vi "DecodeRobotsVSSwithOrientation.vi"(5 "offset":i32, 7 "error in (no error)":errorcluster, 8 "array w/ subset deleted in":u8[](array[numeric])) -> (0 "error out":errorcluster, 1 "array w/ subset deleted out":u8[](array[numeric]), 3 "Array":T1[](array[typedef]) {"orientation" format="%+4.3f"; "y" format="%+4.3f"; "confidence" format="%4.3f"; "x" format="%+4.3f"})   [LabVIEW 2017]
uses:
  SSL Detection Robot.ctl
  <vilib>/Analysis/Matrix/Datatypes/RealMatrix.ctl
  <vilib>/Analysis/Matrix/NI_Matrix.lvlib
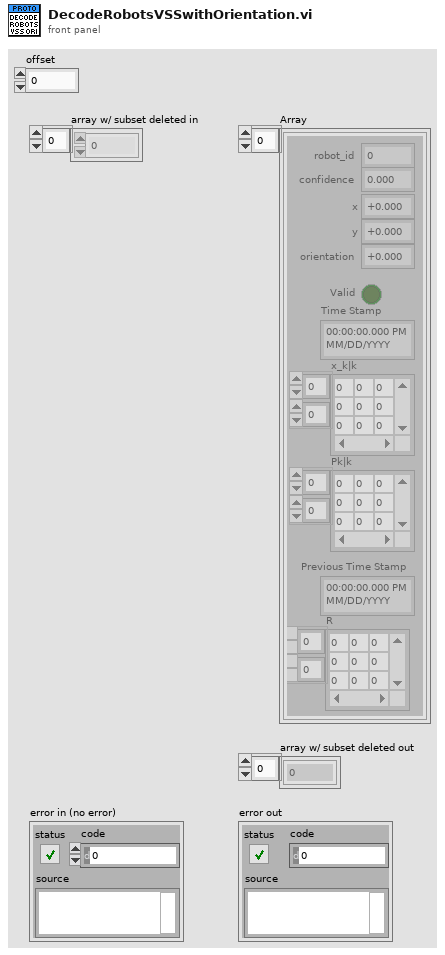
[diagram p1: front panel]
types:
  T1 = typedef "SSL Detection Robot.ctl" = cluster{"x":sgl, "robot_id":u32, "confidence":sgl, "y":sgl, "orientation":sgl, "Valid":bool, "Time Stamp":timestamp, "x_k|k":T2, "Pk|k":T2, "Previous Time Stamp":timestamp, "R":T2}
  T2 = typedef "NI_Matrix.lvlib/RealMatrix.ctl" = dbl[][]
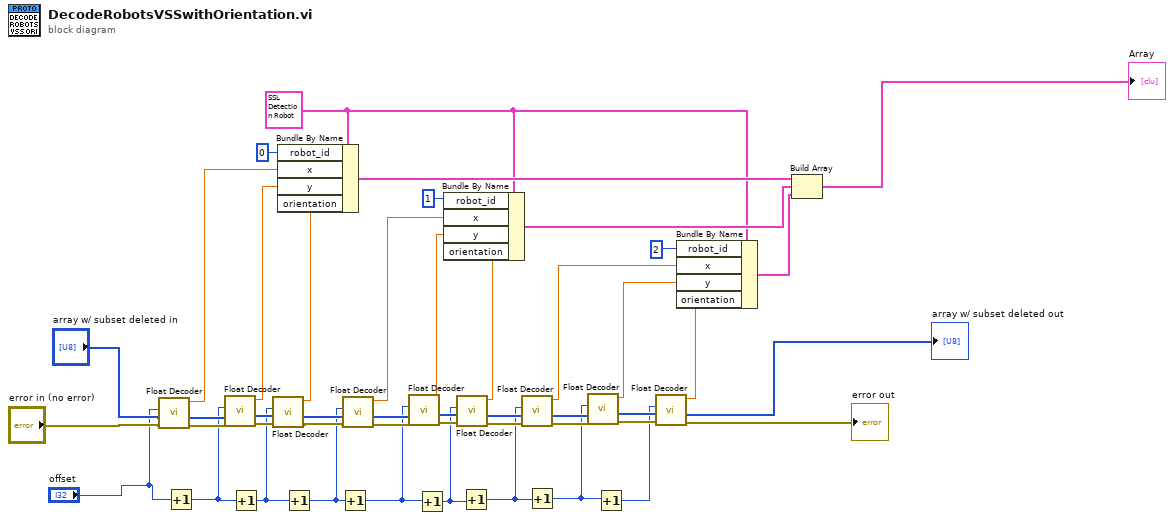
[diagram p0: block diagram]
diagram:
  w39 = T1 {"x"=0.0, "robot_id"=0, "confidence"=0.0, "y"=0.0, "orientation"=0.0, "Valid"=FALSE, "Time Stamp"=timestamp(0 s since 1904-01-01), "x_k|k"=[], "Pk|k"=[], "Previous Time Stamp"=timestamp(0 s since 1904-01-01), "R"=[]} ("element")
  n1 = call "Float Decoder.vi"("error in (no error)"="error in (no error)", "Array"="array w/ subset deleted in", "Key"="offset") -> ("error out"=w15:errorcluster, "array w/ subset deleted"=w14:u8[], "Float"=w13:sgl)  [unwired: 5 in, 1 out]
  n2 = Increment(x="offset") -> (x+1=w9:i32)
  n3 = call "Float Decoder.vi"("error in (no error)"=w15, "Array"=w14, "Key"=w9) -> ("error out"=w16:errorcluster, "array w/ subset deleted"=w17:u8[], "Float"=w18:sgl)  [unwired: 5 in, 1 out]
  n4 = Increment(x=w9) -> (x+1=w8:i32)
  n5 = call "Float Decoder.vi"("error in (no error)"=w16, "Array"=w17, "Key"=w8) -> ("error out"=w25:errorcluster, "array w/ subset deleted"=w24:u8[], "Float"=w19:sgl)  [unwired: 5 in, 1 out]
  n6 = Bundle By Name(cluster=w39, "robot_id"=u32 0, "x"=w13, "y"=w18, "orientation"=w19) -> (w43:T1)
  n7 = Increment(x=w8) -> (x+1=w7:i32)
  n8 = Increment(x=w7) -> (x+1=w6:i32)
  n9 = call "Float Decoder.vi"("error in (no error)"=w25, "Array"=w24, "Key"=w7) -> ("error out"=w22:errorcluster, "array w/ subset deleted"=w23:u8[], "Float"=w27:sgl)  [unwired: 5 in, 1 out]
  n10 = call "Float Decoder.vi"("error in (no error)"=w22, "Array"=w23, "Key"=w6) -> ("error out"=w21:errorcluster, "array w/ subset deleted"=w20:u8[], "Float"=w28:sgl)  [unwired: 5 in, 1 out]
  n11 = Increment(x=w6) -> (x+1=w5:i32)
  n12 = call "Float Decoder.vi"("error in (no error)"=w21, "Array"=w20, "Key"=w5) -> ("error out"=w37:errorcluster, "array w/ subset deleted"=w38:u8[], "Float"=w29:sgl)  [unwired: 5 in, 1 out]
  n13 = Bundle By Name(cluster=w39, "robot_id"=u32 1, "x"=w27, "y"=w28, "orientation"=w29) -> (w42:T1)
  n14 = Increment(x=w5) -> (x+1=w4:i32)
  n15 = call "Float Decoder.vi"("error in (no error)"=w37, "Array"=w38, "Key"=w4) -> ("error out"=w34:errorcluster, "array w/ subset deleted"=w33:u8[], "Float"=w31:sgl)  [unwired: 5 in, 1 out]
  n16 = Increment(x=w4) -> (x+1=w3:i32)
  n17 = call "Float Decoder.vi"("error in (no error)"=w34, "Array"=w33, "Key"=w3) -> ("error out"=w35:errorcluster, "array w/ subset deleted"=w36:u8[], "Float"=w40:sgl)  [unwired: 5 in, 1 out]
  n18 = Increment(x=w3) -> (x+1=w2:i32)
  n19 = call "Float Decoder.vi"("error in (no error)"=w35, "Array"=w36, "Key"=w2) -> ("error out"=→"error out":errorcluster, "array w/ subset deleted"=→"array w/ subset deleted out":u8[], "Float"=w30:sgl)  [unwired: 5 in, 1 out]
  n20 = Bundle By Name(cluster=w39, "robot_id"=u32 2, "x"=w31, "y"=w40, "orientation"=w30) -> (w41:T1)
  n21 = Build Array(w43, w42, w41) -> (→"Array":T1[])
